vi "Change FPGA State.vi"(8 "error in":errorcluster, 11 "cPAS in":refnum<class "cPAS.lvclass">) -> (0 "error out":errorcluster, 3 "cPAS out":refnum<class "cPAS.lvclass">)   [LabVIEW 2015, in "cPAS.lvclass"]
uses:
  cPAS.lvclass
  cPAS.lvclass/cPAS.ctl
  Read Speaker Voltage.vi
  Read FPGA_Ref.vi
  Reusable/PAS/Main/Read Cells.vi
  Reusable/PAS/Main/Get Speaker State.vi
  <vilib>/Utility/error.llb/Error Cluster From Error Code.vi
  <vilib>/rvi/errors/niLvFpgaAdjustHostInterfaceError.vi
  Reusable/PAS/Main/Read Data.vi
  Reusable/PAS/Main/Write Data.vi
  Interface/fpga_ctl.ctl
  Reusable/PAS/Cell/PAS Cell.lvclass
  <vilib>/rvi/interface/nirviReadWriteControl/nirviReadWriteControl.xnode
  Utilities/FPGA/Controls/FxdPt Props.ctl
  Reusable/PAS/Main/Controls/Laser Modulation.ctl
  FPGA Bitfiles/FPGA Server.lvbitx
  Reusable/PAS/Data/Main/PAS Data.lvclass
  NiFpgaLv.dll
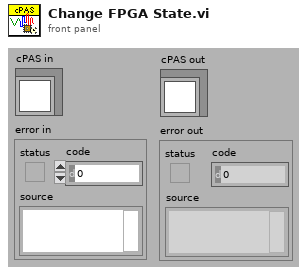
[diagram p1: front panel]
types:
  T1 = typedef "fpga_ctl.ctl" = refnum<k20>
  T2 = typedef "Laser Modulation.ctl" = enum8{"Sine", "Square"}
  T3 = typedef "FxdPt Props.ctl" = cluster{"f0":fxp<+,32,0>, "Scale":fxp<+,14,1>, "Offset":i16, "Mod":T2}
  T4 = cluster{"[0]":bool, "[1]":bool, "[2]":bool, "[3]":bool, "[4]":bool}
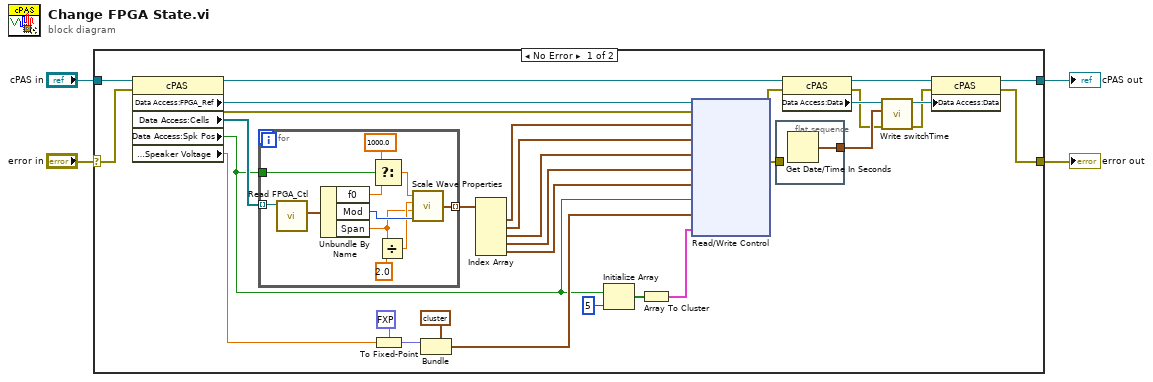
[diagram p0: block diagram]
diagram:
  n1 = case shown="No Error" "error in" {
    selector: "error in" -> [w18 w48]
    tunnel: [w22 w48] -> w3
    tunnel: [w23 w47] -> w1
    tunnel: "cPAS in" -> [w19 w47]
    frame No Error {
      n2 = property class="cPAS"(reference=w19, error in=w18) -> (reference out=w15:refnum<class "cPAS.lvclass">, error out=w14:errorcluster, "Data Access:FPGA_Ref"=w17:T1, "Data Access:Cells"=w16:refnum<class "PAS Cell.lvclass">[], "Data Access:Spk Pos"=w8:bool, "Data Access:Speaker Voltage"=w9:sgl)
      n3 = for {
        tunnel: [w46] -> w34 mode=indexing
        tunnel: w16 -> [w44] mode=indexing
        tunnel: w8 -> [w39]
        n4 = call "Read FPGA_Ctl.vi"("PAS Cell in"=w44) -> ("FPGA_Ctl"=w45:cluster{"Mod":T2, "Span":sgl, "f0":sgl})  [unwired: 8 in, 2 out]
        n5 = Unbundle By Name(w45) -> ("f0"=w38:sgl, "Mod"=w43:T2, "Span"=w40:sgl)
        n6 = Select(t=sgl 1000.0, s=w39, f=w38) -> (s? t:f=w36:sgl)
        n7 = Divide(x=w40, y=sgl 2.0) -> (x/y=w42:sgl)
        n8 = call "Scale Wave Properties.vi"("f0"=w36, "DCoffset"=w42, "Vspan"=w40, "Mod"=w43) -> ("FXP Props"=w46:T3)  [unwired: 1 in]
      }
      n9 = To Fixed-Point(fixed-point type=fxp<+,14,1> 0.0, number=w9) -> (fixed-point=w12:fxp<+,14,1>)
      n10 = Bundle(cluster=cluster{"Voltage":fxp<+,14,1>, "Offset":i16} {"Voltage"=0.0, "Offset"=0} ("Speaker"), "Voltage"=w12) -> (w10:cluster{"Voltage":fxp<+,14,1>, "Offset":i16})  [unwired: 1 in]
      n11 = Index Array(array=w34) -> (element #1=w33:T3, element #2=w32:T3, element #3=w31:T3, element #4=w30:T3, element #5=w29:T3)  [unwired: 5 in]
      n12 = Initialize Array(w8, 5 ("dimension size")) -> (w6:bool[])
      n13 = Array To Cluster(array=w6) -> (cluster=w5:T4)
      n14 = xnode "Read/Write Control"("FPGA VI Reference In"=w17, "error in"=w14, "Cell 1"=w33, "Cell 2"=w32, "Cell 3"=w31, "Cell 4"=w30, "Cell 5"=w29, "Spk Enable"=w8, "Speaker"=w10, "iSpk Enable"=w5) -> ("error out"=w21:errorcluster)  [unwired: 1 out]
      n15 = flat-sequence {
        tunnel: w21 -> [_]
        tunnel: [w35] -> w28
        frame #0 {
          n16 = Get Date/Time In Seconds() -> (seconds since 1Jan1904=w35:timestamp)
        }
      }
      n17 = property class="cPAS"(reference=w15, error in=w21) -> (reference out=w26:refnum<class "cPAS.lvclass">, error out=w20:errorcluster, "Data Access:Data"=w27:refnum<class "PAS Data.lvclass">)
      n18 = call "Write switchTime.vi"("error in (no error)"=w20, "switchTime"=w28, "PAS Data in"=w27) -> ("error out"=w24:errorcluster, "PAS Data out"=w25:refnum<class "PAS Data.lvclass">)  [unwired: 7 in]
      n19 = property class="cPAS"(reference=w26, error in=w24, "Data Access:Data"=w25) -> (reference out=w23:refnum<class "cPAS.lvclass">, error out=w22:errorcluster)
    }
    frame Error {
    }
  }
  "error out" <- w3
  "cPAS out" <- w1
